vi "Set Position.vi"(8 "Error In":errorcluster, 10 "Position":u32, 11 "ByteBuffer In":refnum<class "ByteBuffer.lvclass">) -> (0 "Error Out":errorcluster, 3 "ByteBuffer Out":refnum<class "ByteBuffer.lvclass">)   [LabVIEW 2015, in "ByteBuffer.lvclass"]
doc: "Sets this buffer's position. If the mark is defined and larger than the new position then it is discarded.\n\nParameters:\n+ Position - The new position value, must be non-negative and no larger than the current limit.\n\nReturns:\nThis buffer.\n\nThrows:\n+ IllegalArgumentException - If the preconditions on new position do not hold."
uses:
  ByteBuffer.lvclass
  ByteBuffer.lvclass/ByteBuffer.ctl
  <vilib>/Utility/error.llb/Error Cluster From Error Code.vi
  <vilib>/ErrorRing/Error Ring.xnode
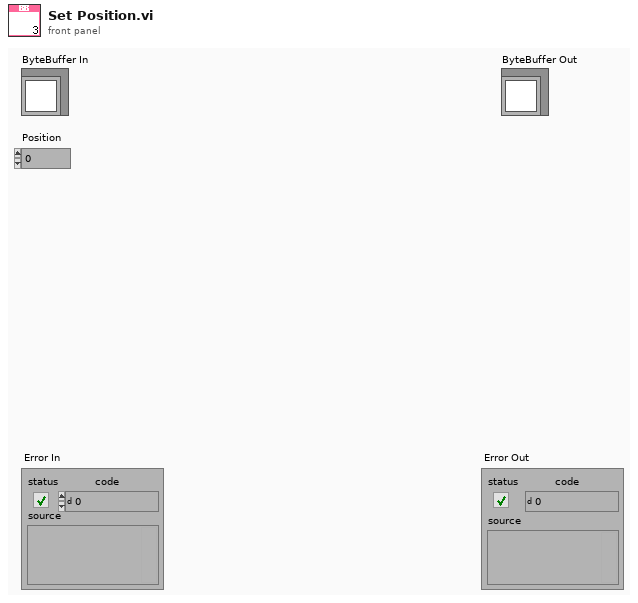
[diagram p1: front panel]
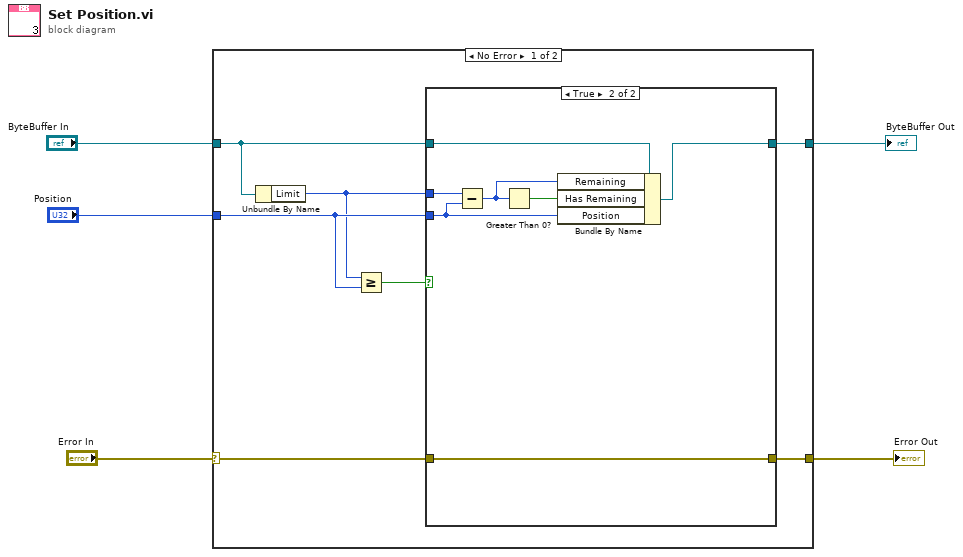
[diagram p0: block diagram]
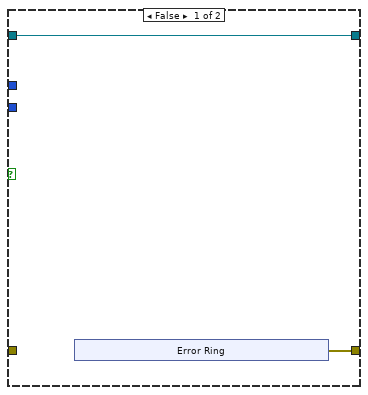
[diagram p2: hidden frame]
diagram:
  n1 = case shown="No Error" "Error In" {
    selector: "Error In" -> [w10 w28]
    tunnel: [w7 w28] -> w4
    tunnel: "ByteBuffer In" -> [w11 w27]
    tunnel: "Position" -> [w8 _]
    tunnel: [w12 w27] -> w1
    frame No Error {
      n2 = Unbundle By Name(w11) -> ("Limit"=w6:u32)
      n3 = Greater Or Equal?(x=w6, y=w8) -> (x >= y?=w9:bool)
      n4 = case shown="True" w9 {
        tunnel: [w14 w26] -> w12
        tunnel: w11 -> [w14 w25]
        tunnel: w10 -> [_ w24]
        tunnel: w8 -> [_ w22]
        tunnel: [w13 w24] -> w7
        tunnel: w6 -> [_ w23]
        frame False {
          n5 = xnode "Error Ring"() -> ("error out"=w13:errorcluster)
        }
        frame True {
          n6 = Subtract(x=w23, y=w22) -> (x-y=w20:u32)
          n7 = Greater Than 0?(x=w20) -> (x > 0?=w21:bool)
          n8 = Bundle By Name(cluster=w25, "Remaining"=w20, "Has Remaining"=w21, "Position"=w22) -> (w26:refnum<class "ByteBuffer.lvclass">)
        }
      }
    }
    frame Error {
    }
  }
  "Error Out" <- w4
  "ByteBuffer Out" <- w1
